vi "Init.vi"(8 "error in (no error)":errorcluster, 11 "Init":bool=TRUE) -> (0 "error out":errorcluster)   [LabVIEW 2020, in "G-Embedded-Python-Interpreter-Toolkit.lvlib"]
uses:
  G-Embedded-Python-Interpreter-Toolkit.lvlib
  bin/gepit.cp310.32.dll
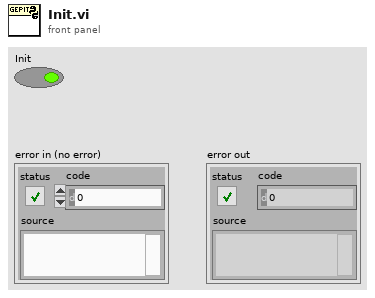
[diagram p1: front panel]
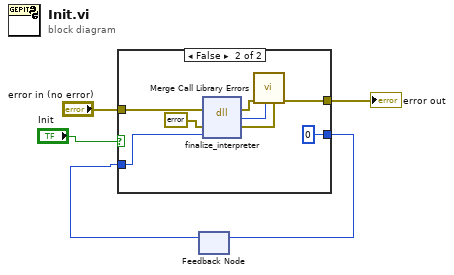
[diagram p0: block diagram]
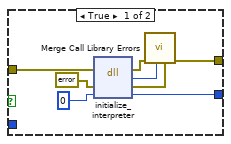
[diagram p2: hidden frame]
diagram:
  n1 = feedback #1() -> (w1:u64)  [unwired: 1 in]
  n2 = case shown="False" "Init" {
    tunnel: [w8 w17] -> w5
    tunnel: "error in (no error)" -> [w7 w16]
    tunnel: w1 -> [_ w15]
    tunnel: [w6 u64 0 ("Session")] -> w3
    frame True {
      n3 = dll-call lib="C:/serenial/libraries/g-embedded-python-interpreter-toolkit/LabVIEW/bin/gepit.cp310.32.dll" fn="initialize_interpreter"(error in=w7, "Error"=errorcluster {"status"=FALSE, "code"=0, "source"=""} ("error constant"), "Session"=u64 0) -> (error out=w11:errorcluster, "return type"=w12:i32, "Error"=w13:errorcluster, "Session"=w6:u64)  [unwired: 2 in, 1 out]
      n4 = call "Merge Call Library Errors.vi"("Call Library Error"=w13, "Return Value"=w12, "error in"=w11) -> ("error out"=w8:errorcluster)  [unwired: 8 in]
    }
    frame False {
      n5 = dll-call lib="C:/serenial/libraries/g-embedded-python-interpreter-toolkit/LabVIEW/bin/gepit.cp310.32.dll" fn="finalize_interpreter"(error in=w16, "Error"=errorcluster {"status"=FALSE, "code"=0, "source"=""} ("error constant"), "Session"=w15) -> (error out=w19:errorcluster, "return type"=w20:i32, "Error"=w21:errorcluster)  [unwired: 3 in, 1 out]
      n6 = call "Merge Call Library Errors.vi"("Call Library Error"=w21, "Return Value"=w20, "error in"=w19) -> ("error out"=w17:errorcluster)  [unwired: 8 in]
    }
  }
  "error out" <- w5
  n7 = feedback-in #1(w3) -> ()
